vi "TSM SSC Digital PPMU Configure Voltage Limits.vi"(0 "Digital TSM In":T1, 5 "Voltage Limit High (V)":dbl=2.5 format="%#_13g", 7 "Voltage Limit Low (V)":dbl=-1.5 format="%#_13g", 11 "error in":errorcluster) -> (4 "Digital TSM Out":T1, 15 "error out":errorcluster)   [LabVIEW 2019]
doc: "Specifies the voltage limit high, or high clamp voltage (VCH), and voltage limit low, or low clamp voltage (VCL) for the specified pins and pin group(s) when forcing current. You must call the PPMU Source VI for changes to the PPMU configuration to take effect, even if the PPMU is already sourcing."
uses:
  TSM/TSM SSC Digital.ctl
  <vilib>/NI_TestStand_SemiconductorModule/NI_TestStand_Semiconductor_Module.lvlibp/PinMap/Digital Pattern/PinQueryContext/DigitalPatternPinQueryContext.lvclass
  SSC Digital/SSC Digital.ctl
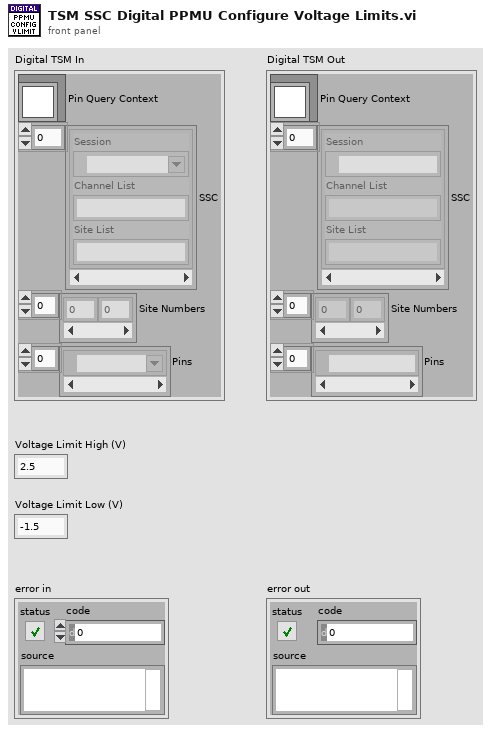
[diagram p1: front panel]
types:
  T1 = typedef "TSM SSC Digital.ctl" = cluster{"Pin Query Context":refnum<class "DigitalPatternPinQueryContext.lvclass">, "SSC":T2[], "Site Numbers":i32[], "Pins":tag[]}
  T2 = typedef "SSC Digital.ctl" = cluster{"Session":refnum<k15>, "Channel List":string, "Site List":string}
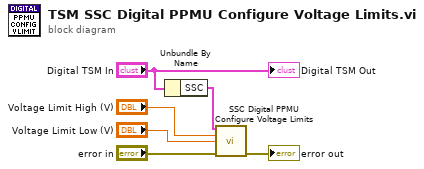
[diagram p0: block diagram]
diagram:
  n1 = Unbundle By Name("Digital TSM In") -> ("SSC"=w5:T2[])
  n2 = call "SSC Digital PPMU Configure Voltage Limits.vi"("Digital SSC in"=w5, "Voltage Limit High (V)"="Voltage Limit High (V)", "Voltage Limit Low (V)"="Voltage Limit Low (V)", "error in"="error in") -> ("error out"=→"error out":errorcluster)  [unwired: 10 in, 1 out]
  "Digital TSM Out" <- "Digital TSM In"
